vi "Initialize Front Panel.vi"(8 "error in (no error)":errorcluster, 11 "Beta View in":refnum<class "Beta View.lvclass">) -> (0 "error out":errorcluster, 3 "Beta View out":refnum<class "Beta View.lvclass">)   [LabVIEW 2017, in "Beta View.lvclass"]
doc: "<License>\nCopyright © 2017 Composed Systems, LLC | All rights reserved\nwww.composed.io\n\nAuthor: Ethan Stern <ethan.stern@composed.io>\n\nThis software is provided \"AS IS\" WITHOUT WARRANTIES, either express or implied, AND IS FOR EDUCATIONAL PURPOSES ONLY.\n</License>"
uses:
  <vilib>/gpm_packages/@cs/popup-viewmanager/Example/Beta View/Beta View.lvclass
  <vilib>/gpm_packages/@cs/popup-viewmanager/Example/Beta View/Beta View.lvclass/Beta View.ctl
  <vilib>/gpm_packages/@cs/mva-viewable/Source/IViewable/IViewable/IViewable.lvclass
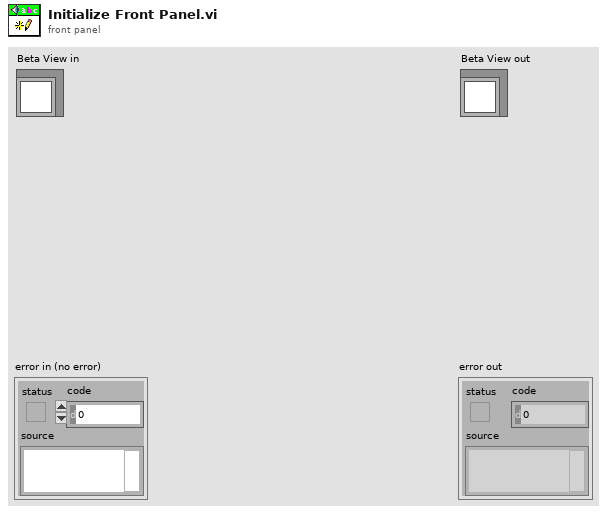
[diagram p1: front panel]
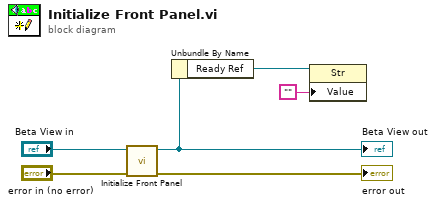
[diagram p0: block diagram]
diagram:
  n1 = call-parent "Initialize Front Panel.vi"("error in (no error)"="error in (no error)", "IViewable in"="Beta View in") -> ("error out"=→"error out":errorcluster, "IViewable out"=w3:refnum<class "Beta View.lvclass">)  [unwired: 8 in]
  "Beta View out" <- w3
  n2 = Unbundle By Name(w3) -> ("Ready Ref"=w1:refnum<vi>)
  n3 = property class="Str"(reference=w1, "Value"="") -> ()  [unwired: 1 in, 2 out]
